vi "CustomGaussianKernel.vi"() -> (2 "array":dbl[][](array[numeric]))   [LabVIEW 2018]
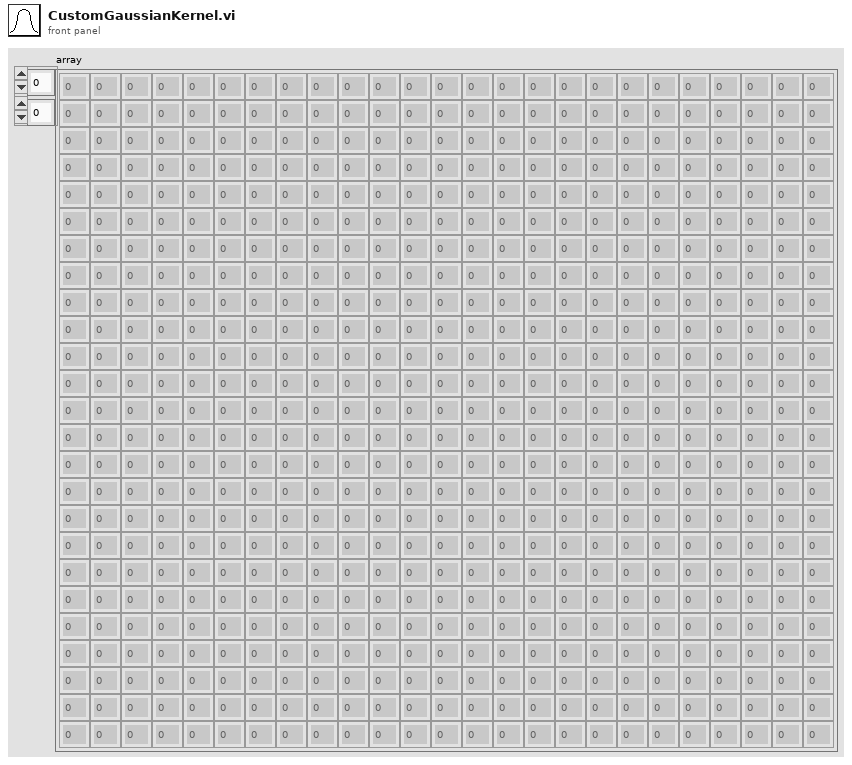
[diagram p1: front panel]
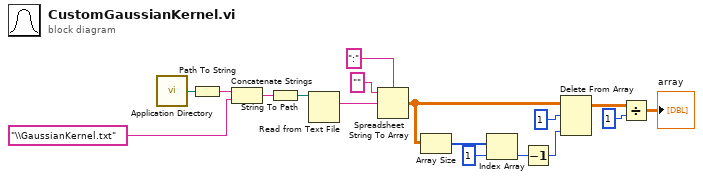
[diagram p0: block diagram]
diagram:
  n1 = call <vilib>:"Application Directory.vi"() -> ("Application Directory"=w5:path)
  n2 = Path To String(path=w5) -> (string=w4:string)
  n3 = Concatenate Strings(w4, "\\GaussianKernel.txt") -> (w1:string)
  n4 = String To Path(string=w1) -> (path=w2:path)
  n5 = Read from Text File(file (use dialog)=w2) -> (text=w9:string)  [unwired: 3 in, 3 out]
  n6 = Spreadsheet String To Array(delimiter (Tab)=":", format string="", spreadsheet string=w9) -> (array=w11:dbl[][])  [unwired: 1 in]
  n7 = Array Size(array=w11) -> (size(s)=w15:i32[])
  n8 = Index Array(array=w15, index=1) -> (element=w13:i32)
  n9 = Decrement(x=w13) -> (x-1=w10:i32)
  n10 = Delete From Array(array=w11, length=1, index (col)=w10) -> (array with subset deleted=w7:dbl[][])  [unwired: 1 in, 1 out]
  n11 = Divide(x=w7, y=1) -> (x/y=→"array":dbl[][])
